vi "Example String Functions 1.vi"(8 "Error In":errorcluster) -> (0 "Error Out":errorcluster)   [LabVIEW 2014]
panel:
  out "offset past match":i32
  out "after substring":string
  out "match substring":string
  out "before substring":string
  out "substring":string
  out "length":i32
  out "concatenated string 2":string
  out "concatenated string":string
  out "all lower case string":string
  out "all upper case string":string
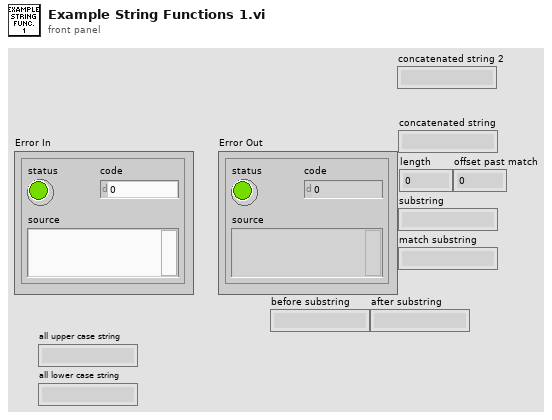
[diagram p1: front panel]
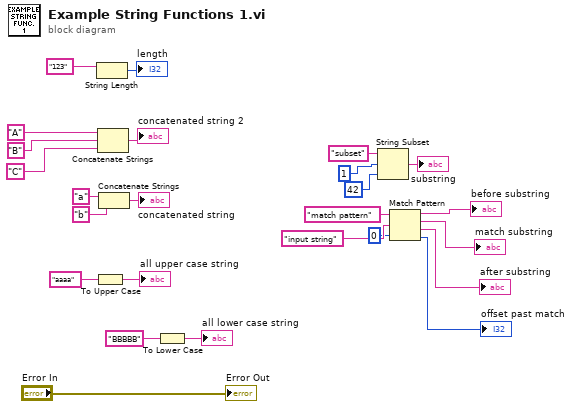
[diagram p0: block diagram]
diagram:
  n1 = To Upper Case(1:"aaaa" ("string")) -> (0:→"all upper case string":string)
  n2 = String Length(string="123") -> (length=→"length":i32)
  n3 = Concatenate Strings("A" ("string"), "B" ("string"), "C" ("string")) -> (→"concatenated string 2":string)
  n4 = Concatenate Strings("a" ("string"), "b" ("string")) -> (→"concatenated string":string)
  n5 = To Lower Case(string="BBBBB") -> (all lower case string=→"all lower case string":string)
  n6 = String Subset(string="subset", offset (0)=1, length (rest)=42 ("length (rest)")) -> (substring=→"substring":string)
  n7 = Match Pattern(string="match pattern", regular expression="input string", offset (0)=0) -> (before substring=→"before substring":string, match substring=→"match substring":string, after substring=→"after substring":string, offset past match=→"offset past match":i32)
  "Error Out" <- "Error In"
